vi "DMSC.main.vi"() -> ()   [LabVIEW 2014, in "DMSClient.lvlib"]
doc: "This CS tool subscribes to the following information of a CS controls domain.\n\n \"DOMAINNAME_Tasks@NODENAME\": A list of taks. Each task has a name, command line parameters and options. There is one service for each node.\n\nHistory: 16-FEB-2006, Dietrich Beck\n\nCopyright (C)\nGesellschaft für Schwerionenforschung, GSI\nPlanckstr. 1\n64291 Darmstadt\nGermany\n\nContact: D.Beck@gsi.de \n\nThis program is free software; you can redistribute it and/or modify it under the terms of the \nGNU General Public License as published by the Free Software Foundation; either version 2 of the license, or (at your option) any later version.\n\nThis program is distributed in the hope that it will be useful, but WITHOUT ANY WARRANTY; without even the implied warranty of MERCHANTABILITY or FITNESS FOR A PARTICULAR PURPOSE. See the GNU General License for more details (http://www.gnu.org).\n\nGesellschaft für Schwerionenforschung, GSI\nPlanckstr. 1, 64291 Darmstadt, Germany\nFor all questions and ideas contact D. Beck.\nLast update: 16-DEC-2005"
uses:
  DMSClient.lvlib
  DMSC.node_type.ctl
  DomainManagementUtils/DMSU.restart_mode.ctl
  DMSC.process_type.ctl
  CSlibraries/UtilityLib/UtilityLib.valueStatus.ctl
  CSlibraries-extern/DimLVEvent/LVDimInterface/LVDimInterface.dim service type.ctl
  <vilib>/Utility/config.llb/Read Key (Boolean).vi
  CSlibraries-extern/DimLVEvent/LVDimInterface/LVDimInterface.dic_info_service_notifier.vi
  CSlibraries-extern/DimLVEvent/LVDimInterface/LVDimInterface.lvlib
  CSlibraries-extern/DimLVEvent/NodeMon-LV/LVNodeInfo/LVNodeInfo.lvlib
  DomainManagementUtils/DMSUtils.lvlib
  CSlibraries/UtilityLib/UtilityLib.lvlib
  <vilib>/Utility/config.llb/NI_LVConfig.lvlib
panel:
  in  "PlaceHolder":bool
  out "myTasks":T1 {"processes"."restartMode" items=["UNKNOWN", "MANUAL", "ONCE", "ALWAYS", "KILL", "SHUTDOWN"]}
  in  "Messages":i32(listbox)
  in  "DMSSNode":string="DMSNode"
  in  "setDomain":bool
  in  "ProcessType":T3 {"restartMode" items=["UNKNOWN", "MANUAL", "ONCE", "ALWAYS", "KILL", "SHUTDOWN"]}
  in  "procTypeArr":T3[](array[typedef]) {"restartMode" items=["UNKNOWN", "MANUAL", "ONCE", "ALWAYS", "KILL", "SHUTDOWN"]}
  in  "DomainName":string="KSTest"
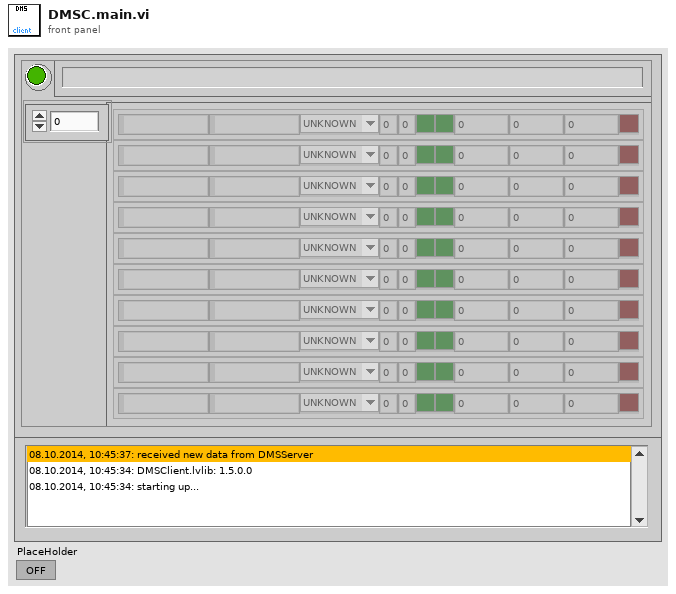
[diagram p1: front panel]
types:
  T1 = typedef "DMSClient.lvlib/DMSC.node_type.ctl" = cluster{"nodeName":string, "processes":cluster{"imageName":string, "argumentString":string, "restartMode":T2, "nOfRestart":i32, "resetRestartTimer":i32, "killOnExit":bool, "csSystem":bool, "PID":dbl, "PMem":dbl, "CPUTime":dbl, "startCnt":i32, "startTime":u32, "restartFailed":bool}[], "no link":bool}
  T2 = typedef "DMSUtils.lvlib/DMSU.restart_mode.ctl" = u16
  T3 = typedef "DMSClient.lvlib/DMSC.process_type.ctl" = cluster{"imageName":string, "argumentString":string, "restartMode":T2, "nOfRestart":i32, "resetRestartTimer":i32, "killOnExit":bool, "csSystem":bool, "PID":dbl, "PMem":dbl, "CPUTime":dbl, "startCnt":i32, "startTime":u32, "restartFailed":bool}
  T4 = cluster{"Command":enum16{"NewSystem", "DestroySystem", "SDSystem"}, "SystemName":string}
  T5 = enum32{"Invalid", "Standard", "Closed", "Hidden", "Minimized", "Maximized"}
  T6 = typedef "UtilityLib.lvlib/UtilityLib.valueStatus.ctl" = enum16{"no info available", "stand by/off", "on", "warning", "alarm/malfunction", "not implemented", "user action required", "important information", "system default", "control default", "indicator default", "button default"}
  T7 = enum16{"AddMessage", "AddErrorMessage", "GetMessages"}
  T8 = enum32{"invalid app kind", "Development System", "Run Time System", "Student Edition", "Embedded LabVIEW", "Evaluation", "Custom"}
  T9 = typedef "NI_LVConfig.lvlib/Config Data RefNum.ctl" = refnum<k1>
  T10 = typedef "LVDimInterface.lvlib/LVDimInterface.dim service type.ctl" = u16
  T11 = cluster{"imageName":string, "argumentString":string, "restartMode":T2, "nOfRestart":i32, "resetRestartTimer":i32, "killOnExit":bool, "csSystem":bool, "PID":dbl, "PMem":dbl, "CPUTime":dbl, "startCnt":i32, "startTime":u32, "restartFailed":bool}[]
  T12 = cluster{"imageName":string, "argumentString":string, "restartMode":T2, "nOfRestart":i32, "resetRestartTimer":i32, "killOnExit":bool, "csSystem":bool, "PID":dbl, "PMem":dbl, "CPUTime":dbl, "startCnt":i32, "startTime":u32, "restartFailed":bool}
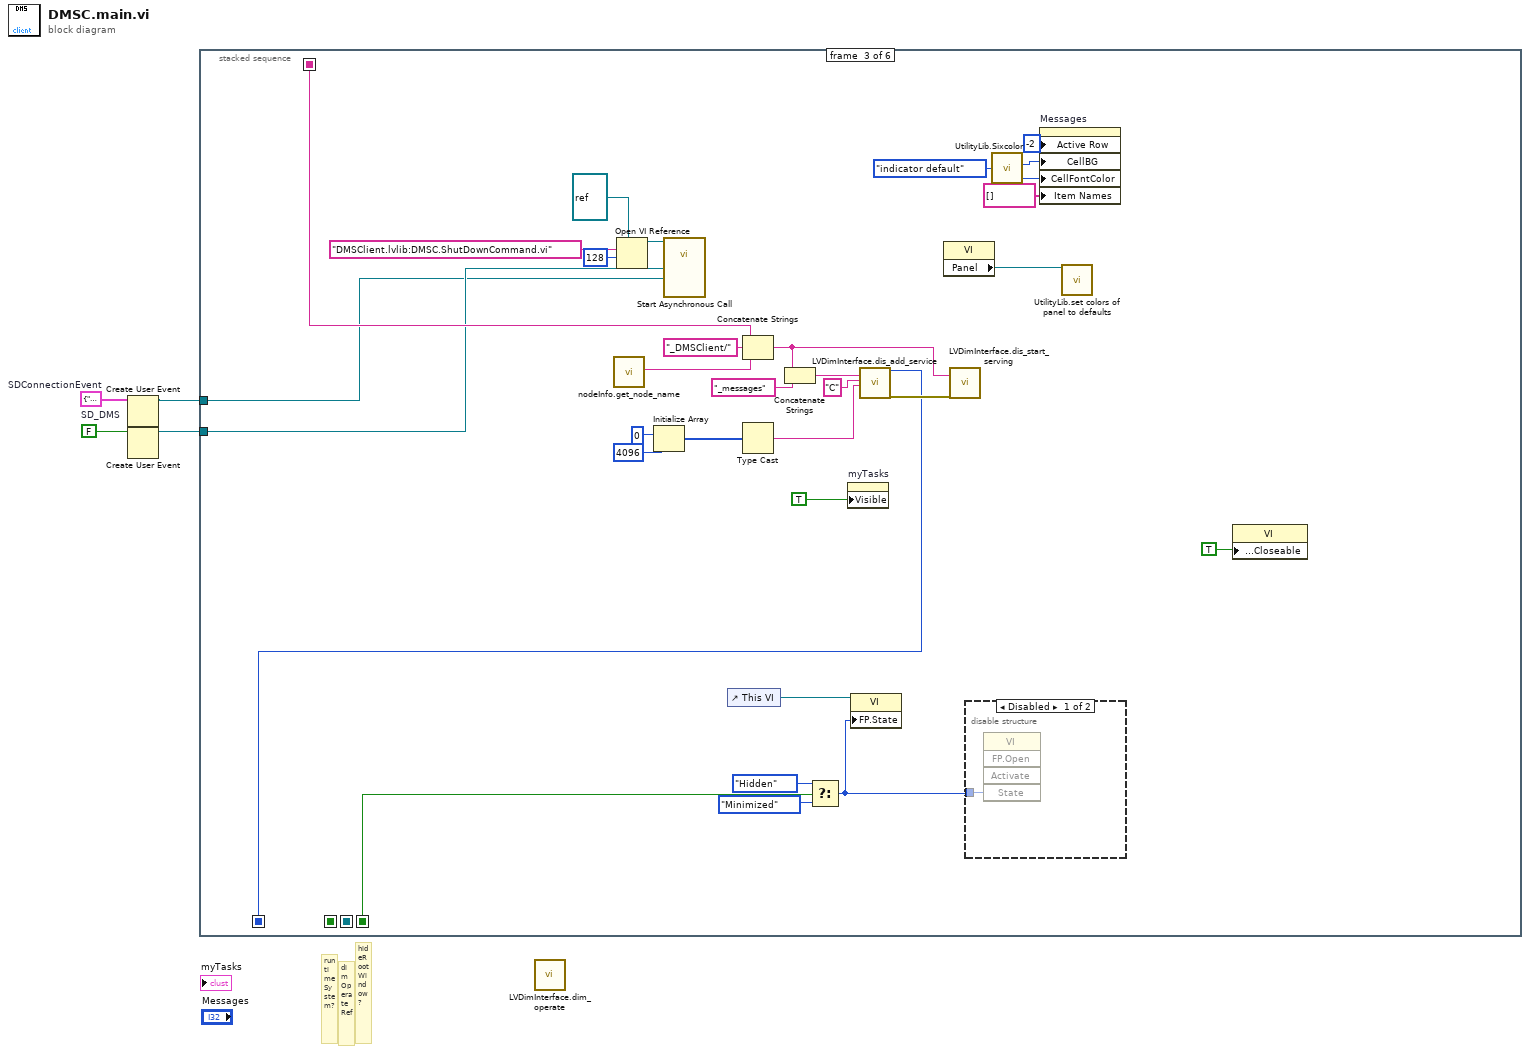
[diagram p0: block diagram]
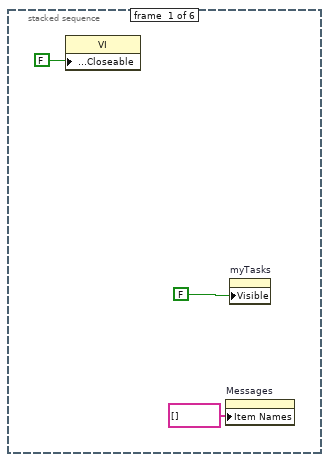
[diagram p2: hidden frame]
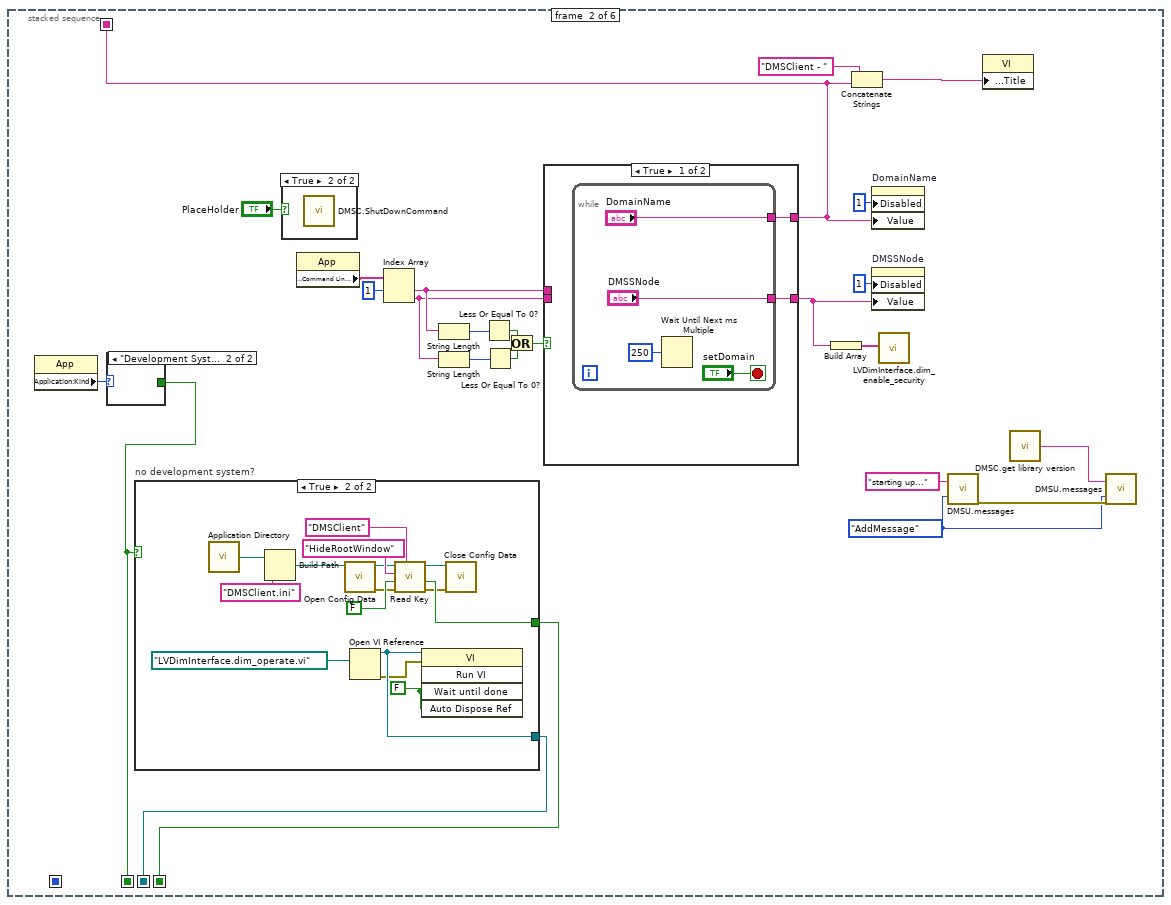
[diagram p3: hidden frame]
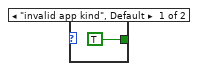
[diagram p5: hidden frame]
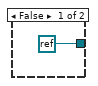
[diagram p6: hidden frame]
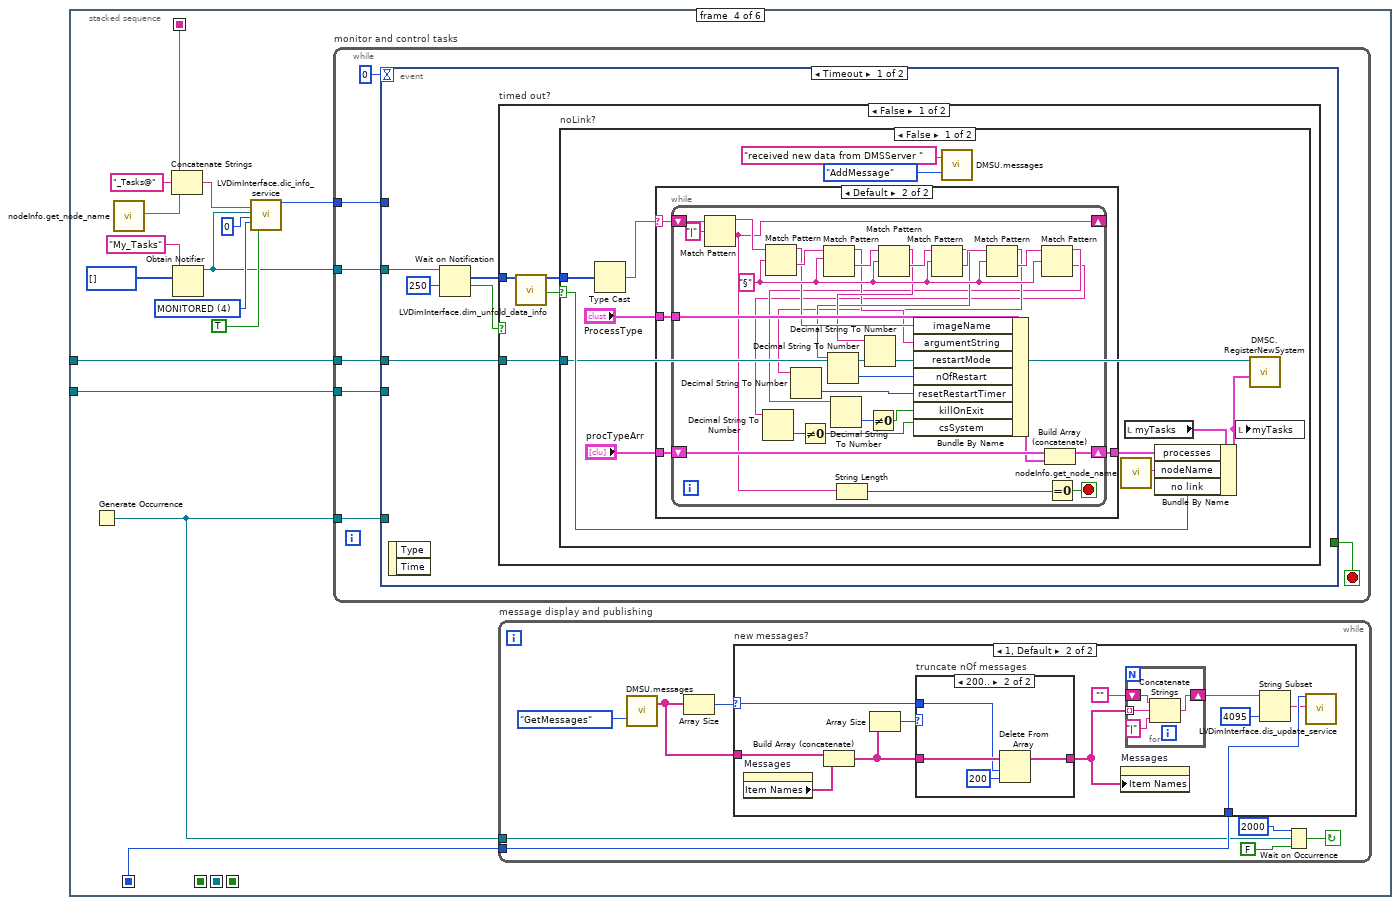
[diagram p9: hidden frame]
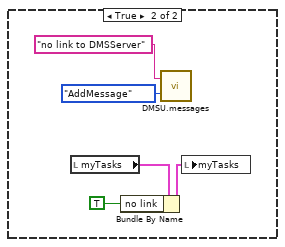
[diagram p13: hidden frame]
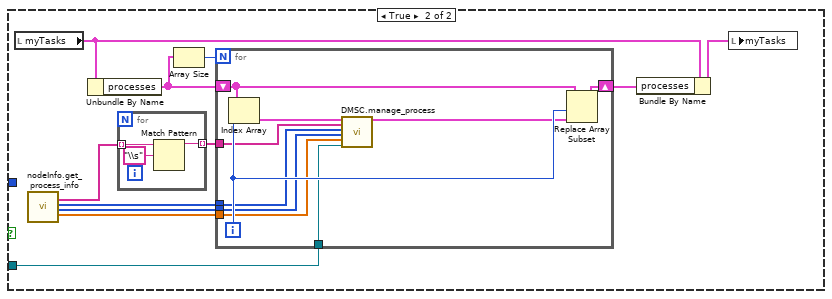
[diagram p14: hidden frame]
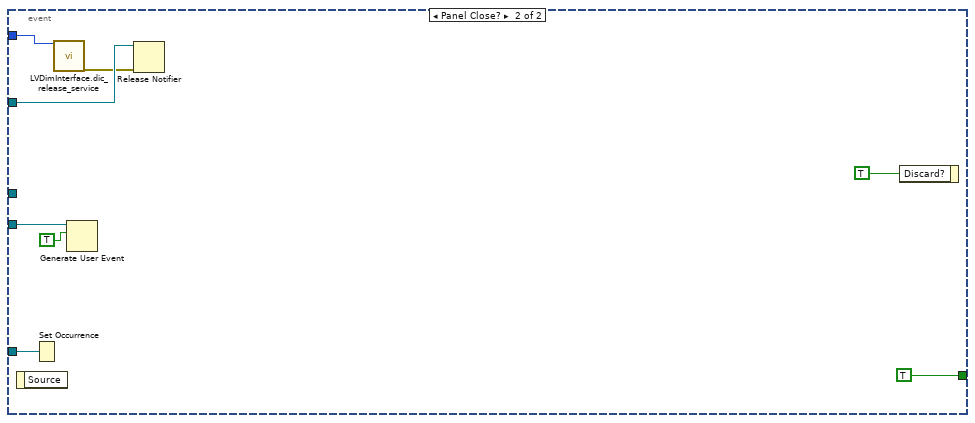
[diagram p15: hidden frame]
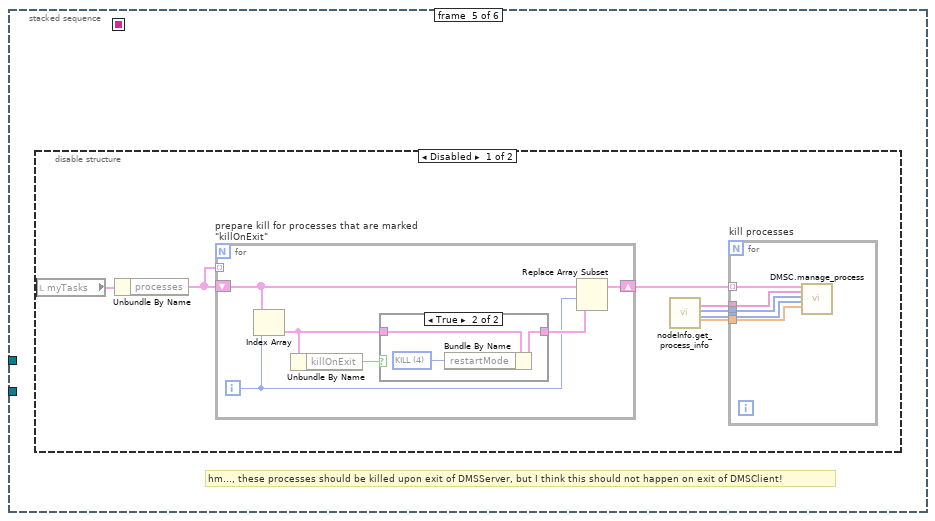
[diagram p16: hidden frame]
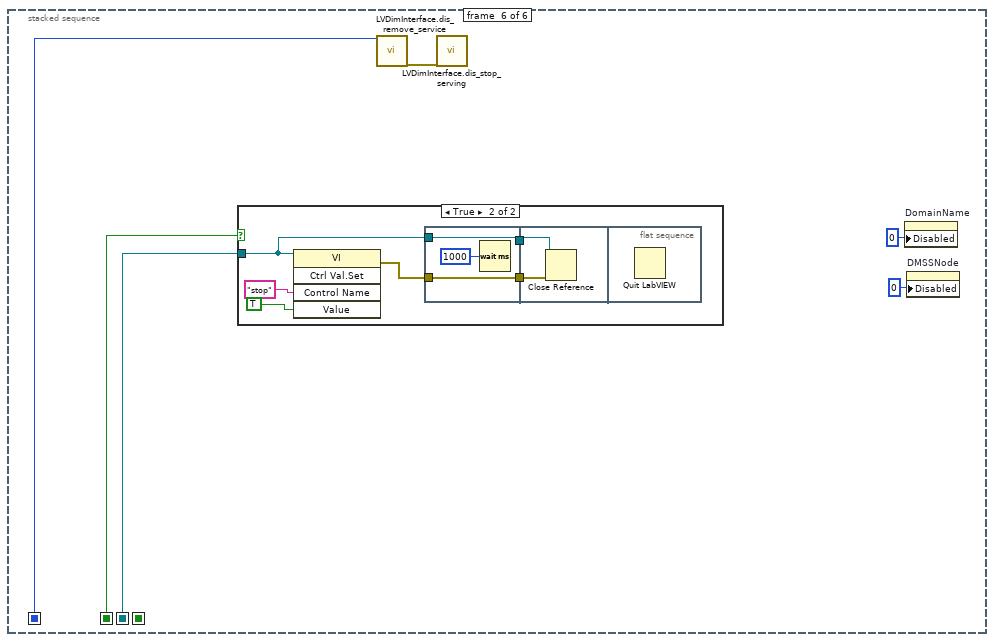
[diagram p19: hidden frame]
diagram:
  w3 = T4 {"Command"=enum."NewSystem", "SystemName"=""}  # SDConnectionEvent
  w4 = FALSE  # SD_DMS
  # "hideRootWindow?"
  # "dimOperateRef"
  # "runtimeSystem?"
  n1 = Create User Event(user event datatype=w3) -> (user event=w2:refnum<user-event>)  [unwired: 1 in, 1 out]
  n2 = Create User Event(user event datatype=w4) -> (user event=w1:refnum<user-event>)  [unwired: 1 in, 1 out]
  n3 = stacked-sequence {
    seq-local: [_ w15 _ _ _ _] -> [_ _ w76 w105 _ _]
    seq-local: [_ w17 _ _ _ _] -> [_ _ _ _ _ w256]
    seq-local: [_ w19 _ _ _ _] -> [_ _ _ _ _ w257]
    seq-local: [_ _ w77 _ _ _] -> [_ _ _ w94 _ w258]
    seq-local: [_ w12 _ _ _ _] -> [_ _ w64 _ _ _]
    tunnel: w2 -> [_ _ w60 w92 _ _]
    tunnel: w1 -> [_ _ w61 w91 _ _]
    frame #0 {
      n4 = property class="VI"("Front Panel.Closeable"=FALSE ("Front Panel Window:Closeable")) -> ()  [unwired: 2 in, 2 out]
      n5 = property on="Messages" class="LstBox (strict)"("Item Names"=string[] []) -> ()  [unwired: 2 in, 2 out]
      n6 = property on="myTasks" class="Clust (strict)"("Visible"=FALSE) -> ()  [unwired: 2 in, 2 out]
    }
    frame #1 {
      w9 = T7."AddMessage" ("Action")
      n7 = property on="Property Node" class="App"() -> ("Application:Kind"=w18:T8)  [unwired: 2 in, 2 out]
      n8 = case shown="\"Development System\"" w18 {
        tunnel: [TRUE _] -> w17
        frame "invalid app kind", Default {
        }
        frame "Development System" {
        }
      }
      n9 = case "no development system?" shown="True" w17 {
        tunnel: [refnum<k0> refnum ("Not a Refnum Constant") w47] -> w19
        tunnel: [_ w45] -> w12
        frame False {
        }
        frame True {
          w48 = FALSE ("Wait until done")
          n10 = call <vilib>:"Application Directory.vi"() -> ("Application Directory"=w35:path)
          n11 = Build Path(base path=w35, name or relative path="DMSClient.ini") -> (appended path=w36:path)
          n12 = call <vilib>:"Open Config Data.vi"("configuration file path"=w36) -> ("error out"=w38:errorcluster, "refnum"=w41:T9)  [unwired: 8 in, 1 out]
          n13 = Open VI Reference(vi path=path "LVDimInterface.dim_operate.vi") -> (vi reference=w47:refnum<vi>, error out=w46:errorcluster)  [unwired: 5 in]
          n14 = call-poly <vilib>:"Read Key.vi"("section"="DMSClient", "error in (no error)"=w38, "default value"=FALSE, "key"="HideRootWindow", "refnum"=w41) -> ("error out"=w37:errorcluster, "value"=w45:bool, "refnum out"=w40:T9)  [unwired: 3 in, 1 out]
          n15 = invoke on="Invoke Node" class="VI" method="Run VI"(reference=w47, error in=w46, "Wait until done"=w48, "Auto Dispose Ref"=w48) -> ()  [unwired: 1 in, 5 out]
          n16 = call <vilib>:"Close Config Data.vi"("error in (no error)"=w37, "refnum"=w40) -> ()  [unwired: 8 in, 2 out]
        }
      }
      n17 = case shown="True" "PlaceHolder" {
        frame False {
        }
        frame True {
          n18 = call "DMSC.ShutDownCommand.vi"() -> ()  [unwired: 20 in]
        }
      }
      n19 = property on="Property Node" class="App"() -> ("Application:Command Line Arguments"=w32:string[])  [unwired: 2 in, 2 out]
      n20 = Index Array(array=w32, index #1=1 ("index")) -> (element #1=w29:string, element #2=w23:string)  [unwired: 1 in]
      n21 = String Length(string=w29) -> (length=w30:i32)
      n22 = String Length(string=w23) -> (length=w27:i32)
      n23 = Less Or Equal To 0?(x=w30) -> (x <= 0?=w24:bool)
      n24 = Less Or Equal To 0?(x=w27) -> (x <= 0?=w25:bool)
      n25 = Or(x=w24, y=w25) -> (x .or. y?=w26:bool)
      n26 = case shown="True" w26 {
        tunnel: [w51 w57] -> w15
        tunnel: w29 -> [_ w57]
        tunnel: [w50 w56] -> w20
        tunnel: w23 -> [_ w56]
        frame True {
          n27 = while {
            tunnel: ["DomainName"] -> w51
            tunnel: ["DMSSNode"] -> w50
            stop <- "setDomain" stop-if-true
            n28 = Wait Until Next ms Multiple(millisecond multiple=u32 250) -> ()  [unwired: 1 out]
          }
        }
        frame False {
        }
      }
      n29 = Build Array(w20) -> (w21:string[])
      n30 = Concatenate Strings("DMSClient - " ("string"), w15) -> (w13:string)
      n31 = property on="DomainName" class="Str"("Disabled"=u8 1, "Value"=w15) -> ()  [unwired: 2 in, 2 out]
      n32 = property on="DMSSNode" class="Str"("Disabled"=u8 1, "Value"=w20) -> ()  [unwired: 2 in, 2 out]
      n33 = call "LVDimInterface.dim_enable_security.vi"("allowedNodes"=w21) -> ()  [unwired: 18 in, 1 out]
      n34 = call "DMSU.messages.vi"("message"="starting up...", "Action"=w9) -> ("error out"=w11:errorcluster)  [unwired: 16 in, 1 out]
      n35 = property on="Property Node" class="VI"("Front Panel.Title"=w13) -> ()  [unwired: 2 in, 2 out]
      n36 = call "DMSC.get library version.vi"() -> ("nameAndVersion"=w10:string)  [unwired: 1 in]
      n37 = call "DMSU.messages.vi"("message"=w10, "Action"=w9, "error in (no error)"=w11) -> ()  [unwired: 15 in, 2 out]
    }
    frame #2 {
      n38 = call "nodeInfo.get_node_name.vi"() -> ("nodeName"=w83:string)  [unwired: 18 in, 1 out]
      n39 = Open VI Reference(type specifier VI Refnum (for type only)=refnum<vi> refnum, vi path="DMSClient.lvlib:DMSC.ShutDownCommand.vi", options=128) -> (vi reference=w58:refnum<vi>)  [unwired: 3 in, 1 out]
      n40 = Initialize Array(u8 0, 4096 ("dimension size")) -> (w79:u8[])
      n41 = call-by-ref "Start Asynchronous Call"(reference=w58, "SD_DMS"=w61, "SDConnection Event"=w60) -> ()  [unwired: 19 in, 2 out]
      n42 = control-ref of="This VI"() -> (w66:refnum<vi>)
      n43 = Concatenate Strings(w76, "_DMSClient/" ("string"), w83) -> (w86:string)
      n44 = Type Cast(x=w79) -> (*(type *) &x=w78:string)  [unwired: 1 in]
      n45 = Concatenate Strings(w86, "_messages" ("string")) -> (w87:string)
      n46 = Select(t=T5."Hidden", s=w64, f=T5."Minimized" ("State")) -> (s? t:f=w65:T5)
      n47 = property on="myTasks" class="Clust (strict)"("Visible"=TRUE) -> ()  [unwired: 2 in, 2 out]
      n48 = property class="VI"(reference=w66, "FP.State"=w65) -> ()  [unwired: 1 in, 2 out]
      n49 = call "LVDimInterface.dis_add_service.vi"("serviceName"=w87, "typeDescriptor"="C", "data"=w78) -> ("my_serviceID"=w77:i32, "error out"=w85:errorcluster)  [unwired: 15 in]
      n50 = property on="Property Node" class="VI"() -> ("Panel"=w70:refnum<vi>)  [unwired: 2 in, 2 out]
      n51 = call "LVDimInterface.dis_start_serving.vi"("serverName"=w86, "error in (no error)"=w85) -> ()  [unwired: 16 in, 2 out]
      n52 = disable-structure shown="Disabled" {
        disable-tunnel: w65 -> [w90 _]
        frame Disabled {
          n53 = invoke on="Invoke Node" class="VI" method="FP.Open"("State"=w90) -> ()  [unwired: 4 in, 5 out]
        }
        frame Enabled {
        }
      }
      n54 = call "UtilityLib.Sixcolor.vi"("State"=UtilityLib.valueStatus."indicator default") -> ("elementBackground"=w74:u32, "elementText"=w73:u32)  [unwired: 2 in, 2 out]
      n55 = property on="Messages" class="LstBox (strict)"("Active Row"=-2 ("Active Row:Active Row Number"), "CellBG"=w74, "CellFontColor"=w73, "Item Names"=string[] []) -> ()  [unwired: 2 in, 2 out]
      n56 = call "UtilityLib.set colors of panel to defaults.vi"("Front Panel"=w70) -> ()  [unwired: 18 in, 1 out]
      n57 = property class="VI"("Front Panel.Closeable"=TRUE ("Front Panel Window:Closeable")) -> ()  [unwired: 2 in, 2 out]
    }
    frame #3 {
      w98 = T10 4 items=["ONCE_ONLY"=1, "TIMED"=2, "MONITORED"=4] ("serviceType")
      n58 = Generate Occurrence() -> (w93:refnum<k4>)
      n59 = call "nodeInfo.get_node_name.vi"() -> ("nodeName"=w104:string)  [unwired: 18 in, 1 out]
      n60 = Concatenate Strings(w105, "_Tasks@" ("string"), w104) -> (w102:string)
      n61 = Obtain Notifier(name (unnamed)="My_Tasks", notification data type=i8[] []) -> (notifier out=w95:refnum<notifier>)  [unwired: 2 in, 2 out]
      n62 = call-poly "LVDimInterface.dic_info_service.vi"("serviceName"=w102, "notifierRef"=w95, "timeout [s]"=0, "serviceType"=w98, "stamped"=TRUE) -> ("callBackID"=w96:i32)  [unwired: 13 in, 1 out]
      n63 = while "monitor and control tasks" {
        tunnel: w96 -> [w138]
        tunnel: w95 -> [w137]
        tunnel: w93 -> [w136]
        tunnel: w92 -> [w135]
        tunnel: w91 -> [w134]
        stop <- w139 stop-if-true
        n64 = event shown="[0] Timeout" {
          selector: _ -> [_ _]
          dyn-events: _ -> [_ _]
          timeout: 0 -> [_ _]
          tunnel: [_ TRUE ("Discard?")] -> w139
          tunnel: w138 -> [_ w233]
          tunnel: w137 -> [w145 w232]
          tunnel: w136 -> [_ w228]
          tunnel: w135 -> [w141 _]
          tunnel: w134 -> [_ w227]
          event Timeout {
            n65 = event-data() -> ()  [unwired: 1 in, 2 out]
            n66 = Wait on Notification(notifier=w145, timeout in ms (-1)=250) -> (notification=w144:i8[], timed out?=w143:bool)  [unwired: 2 in, 2 out]
            n67 = case "timed out?" shown="False" w143 {
              tunnel: w144 -> [w149 _]
              tunnel: w141 -> [w146 w202]
              frame False {
                n68 = call "LVDimInterface.dim_unfold_data_info.vi"("rawData"=w149) -> ("data"=w147:i8[], "no link"=w148:bool)  [unwired: 8 in, 9 out]
                n69 = case "noLink?" shown="False" w148 {
                  selector: w148 -> [w152 _]
                  tunnel: w147 -> [w161 _]
                  tunnel: w146 -> [w151 _]
                  frame False {
                    n70 = Type Cast(x=w161) -> (*(type *) &x=w153:string)  [unwired: 1 in]
                    n71 = case shown="Default" w153 {
                      selector: w153 -> [_ w163]
                      tunnel: "procTypeArr" -> [w162 w166]
                      tunnel: "ProcessType" -> [_ w165]
                      tunnel: [w162 w164] -> w156
                      frame "noTask" {
                      }
                      frame Default {
                        n72 = while {
                          shift-right: [w170] -> _
                          shift-left: w163 -> [w167]
                          shift-right: [w185] -> w164
                          shift-left: w166 -> [w186]
                          tunnel: w165 -> [w188]
                          stop <- w169 stop-if-true
                          w189 = "§" ("regular expression")
                          n73 = Match Pattern(string=w167, regular expression="|") -> (before substring=w195:string, after substring=w170:string)  [unwired: 1 in, 2 out]
                          n74 = Match Pattern(string=w195, regular expression=w189) -> (before substring=w187:string, after substring=w194:string)  [unwired: 1 in, 2 out]
                          n75 = Match Pattern(string=w194, regular expression=w189) -> (before substring=w179:string, after substring=w193:string)  [unwired: 1 in, 2 out]
                          n76 = String Length(string=w170) -> (length=w168:i32)
                          n77 = Match Pattern(string=w193, regular expression=w189) -> (before substring=w182:string, after substring=w192:string)  [unwired: 1 in, 2 out]
                          n78 = Decimal String To Number(string=w182) -> (number=w183:i32)  [unwired: 2 in, 1 out]
                          n79 = Match Pattern(string=w192, regular expression=w189) -> (before substring=w180:string, after substring=w191:string)  [unwired: 1 in, 2 out]
                          n80 = Decimal String To Number(string=w180) -> (number=w181:i32)  [unwired: 2 in, 1 out]
                          n81 = Match Pattern(string=w191, regular expression=w189) -> (before substring=w178:string, after substring=w190:string)  [unwired: 1 in, 2 out]
                          n82 = Decimal String To Number(string=w178) -> (number=w177:i32)  [unwired: 2 in, 1 out]
                          n83 = Match Pattern(string=w190, regular expression=w189) -> (before substring=w176:string, after substring=w171:string)  [unwired: 1 in, 2 out]
                          n84 = Decimal String To Number(string=w171) -> (number=w173:i32)  [unwired: 2 in, 1 out]
                          n85 = Not Equal To 0?(x=w173) -> (x != 0?=w172:bool)
                          n86 = Decimal String To Number(string=w176) -> (number=w175:i32)  [unwired: 2 in, 1 out]
                          n87 = Not Equal To 0?(x=w175) -> (x != 0?=w174:bool)
                          n88 = Bundle By Name(cluster=w188, "imageName"=w187, "argumentString"=w179, "restartMode"=w183, "nOfRestart"=w181, "resetRestartTimer"=w177, "killOnExit"=w174, "csSystem"=w172) -> (w184:T3)
                          n89 = Build Array (concatenate)(w186, w184) -> (w185:T3[])
                          n90 = Equal To 0?(x=w168) -> (x = 0?=w169:bool)
                        }
                      }
                    }
                    n91 = call "DMSU.messages.vi"("message"="received new data from DMSServer " ("string"), "Action"=T7."AddMessage") -> ()  [unwired: 16 in, 2 out]
                    n92 = call "nodeInfo.get_node_name.vi"() -> ("nodeName"=w157:string)  [unwired: 18 in, 1 out]
                    n93 = local read "myTasks"() -> (w158:T1)
                    n94 = Bundle By Name(cluster=w158, "processes"=w156, "nodeName"=w157, "no link"=w152) -> (w150:T1)
                    n95 = local write "myTasks"(w150) -> ()
                    n96 = call "DMSC.RegisterNewSystem.vi"("myTasks"=w150, "SDConnectionEvent"=w151) -> ()  [unwired: 10 in]
                  }
                  frame True {
                    n97 = local read "myTasks"() -> (w199:T1)
                    n98 = Bundle By Name(cluster=w199, "no link"=TRUE) -> (w198:T1)
                    n99 = call "DMSU.messages.vi"("message"="no link to DMSServer", "Action"=T7."AddMessage") -> ()  [unwired: 16 in, 2 out]
                    n100 = local write "myTasks"(w198) -> ()
                  }
                }
              }
              frame True {
                n101 = local read "myTasks"() -> (w207:T1)
                n102 = call "nodeInfo.get_process_info.vi"() -> ("procNames"=w203:string[], "procID"=w212:i32[], "procMemory"=w211:i32[], "procRuntime"=w210:dbl[])  [unwired: 14 in, 2 out]
                n103 = Unbundle By Name(w207) -> ("processes"=w208:T11)
                n104 = for {
                  tunnel: [w215] -> w204 mode=indexing
                  tunnel: w203 -> [w214] mode=indexing
                  n105 = Match Pattern(string=w214, regular expression="\\s") -> (before substring=w215:string)  [unwired: 1 in, 3 out]
                }
                n106 = Array Size(array=w208) -> (size(s)=w209:i32)
                n107 = for {
                  N: w209 -> [_]
                  tunnel: w204 -> [w220]
                  tunnel: w212 -> [w219]
                  tunnel: w211 -> [w218]
                  tunnel: w210 -> [w217]
                  shift-right: [w223] -> w206
                  shift-left: w208 -> [w224]
                  tunnel: w202 -> [w216]
                  i -> [w225]
                  n108 = Index Array(array=w224, index=w225) -> (element=w222:T12)
                  n109 = call "DMSC.manage_process.vi"("Process"=w222, "procNames"=w220, "procID"=w219, "procMemory"=w218, "procRuntime"=w217, "SDConnectionEvent"=w216) -> ("Process (out)"=w221:T3)  [unwired: 13 in]
                  n110 = Replace Array Subset(array=w224, new element=w221, index=w225) -> (w223:T11)
                }
                n111 = Bundle By Name(cluster=w207, "processes"=w206) -> (w205:T1)
                n112 = local write "myTasks"(w205) -> ()
              }
            }
          }
          event Panel Close? {
            n113 = event-data() -> ()  [unwired: 1 in, 1 out]
            n114 = Set Occurrence(w228) -> ()
            n115 = call "LVDimInterface.dic_release_service.vi"("callBackID"=w233) -> ("error out"=w231:errorcluster)  [unwired: 18 in]
            n116 = Generate User Event(user event=w227, event data cluster=TRUE ("SD_DMS")) -> ()  [unwired: 2 in, 2 out]
            n117 = Release Notifier(notifier=w232, error in (no error)=w231) -> ()  [unwired: 1 in, 3 out]
            n118 = event-data ("Event Filter Node")("Discard?"=TRUE) -> ()  [unwired: 1 in, 1 out]
          }
        }
      }
      n119 = while "message display and publishing" {
        tunnel: w93 -> [w106]
        tunnel: w94 -> [w107]
        stop <- w110 continue-if-true
        n120 = call "DMSU.messages.vi"("Action"=T7."GetMessages") -> ("messages"=w112:string[])  [unwired: 17 in, 1 out]
        n121 = Array Size(array=w112) -> (size(s)=w111:i32)
        n122 = case "new messages?" shown="1, Default" w111 {
          selector: w111 -> [_ w120]
          tunnel: w112 -> [_ w121]
          tunnel: w107 -> [_ w116]
          frame 0 {
          }
          frame 1, Default {
            n123 = property on="Messages" class="LstBox (strict)"() -> ("Item Names"=w124:string[])  [unwired: 2 in, 2 out]
            n124 = Build Array (concatenate)(w121, w124) -> (w122:string[])
            n125 = Array Size(array=w122) -> (size(s)=w123:i32)
            n126 = case "truncate nOf messages" shown="200.." w123 {
              tunnel: w122 -> [w129 w133]
              tunnel: w120 -> [_ w130]
              tunnel: [w129 w131] -> w119
              frame 0, Default {
              }
              frame 200.. {
                n127 = Delete From Array(array=w133, length=w130, index=200) -> (array with subset deleted=w131:string[])  [unwired: 1 out]
              }
            }
            n128 = property on="Messages" class="LstBox (strict)"("Item Names"=w119) -> ()  [unwired: 2 in, 2 out]
            n129 = for {
              tunnel: w119 -> [w127] mode=indexing
              shift-right: [w125] -> w118
              shift-left: "" ("Empty String Constant") -> [w128]
              n130 = Concatenate Strings(w128, w127, "|" ("string")) -> (w125:string)
            }
            n131 = String Subset(string=w118, length (rest)=4095 ("offset (0)")) -> (substring=w115:string)  [unwired: 1 in]
            n132 = call "LVDimInterface.dis_update_service.vi"("my_serviceID"=w116, "data"=w115) -> ()  [unwired: 15 in, 3 out]
          }
        }
        n133 = Wait on Occurrence(1:FALSE ("ignore previous (T)"), 2:w106, 3:2000 ("ms timeout (-1)")) -> (0:w110:bool)
      }
    }
    frame #4 {
      # "hm..., these processes should be killed upon exit of DMSServer, but I think this should not happen on exit of DMSClient!"
      n134 = disable-structure shown="Disabled" {
        frame Disabled {
          n135 = local read "myTasks"() -> (w240:T1)
          n136 = Unbundle By Name(w240) -> ("processes"=w234:T11)
          n137 = for "prepare kill for processes that are marked \"killOnExit\"" {
            shift-right: [w246] -> w239
            shift-left: w234 -> [w249]
            tunnel: w234 -> [_] mode=indexing
            i -> [w247]
            n138 = Index Array(array=w249, index=w247) -> (element=w250:T12)
            n139 = Unbundle By Name(w250) -> ("killOnExit"=w251:bool)
            n140 = case shown="True" w251 {
              tunnel: w250 -> [w252 w255]
              tunnel: [w252 w253] -> w248
              frame False {
              }
              frame True {
                w254 = T2 4 items=["UNKNOWN", "MANUAL", "ONCE", "ALWAYS", "KILL"] ("restartMode")
                n141 = Bundle By Name(cluster=w255, "restartMode"=w254) -> (w253:T12)
              }
            }
            n142 = Replace Array Subset(array=w249, new element=w248, index=w247) -> (w246:T11)
          }
          n143 = call "nodeInfo.get_process_info.vi"() -> ("procNames"=w238:string[], "procID"=w237:i32[], "procMemory"=w236:i32[], "procRuntime"=w235:dbl[])  [unwired: 14 in, 2 out]
          n144 = for "kill processes" {
            tunnel: w239 -> [w245] mode=indexing
            tunnel: w238 -> [w244]
            tunnel: w237 -> [w243]
            tunnel: w236 -> [w242]
            tunnel: w235 -> [w241]
            n145 = call "DMSC.manage_process.vi"("Process"=w245, "procNames"=w244, "procID"=w243, "procMemory"=w242, "procRuntime"=w241) -> ()  [unwired: 14 in, 1 out]
          }
        }
        frame Enabled {
        }
      }
    }
    frame #5 {
      n146 = case shown="True" w256 {
        tunnel: w257 -> [_ w264]
        frame False {
        }
        frame True {
          n147 = invoke on="Invoke Node" class="VI" method="Ctrl Val.Set"(reference=w264, "Control Name"="stop", "Value"=TRUE) -> (error out=w266:errorcluster)  [unwired: 2 in, 4 out]
          n148 = flat-sequence {
            tunnel: w264 -> [w269]
            tunnel: w266 -> [w270]
            tunnel: [w270] -> w263
            tunnel: [w269] -> w262
            tunnel: w263 -> [w272]
            tunnel: w262 -> [w271]
            frame #0 {
              n149 = Wait (ms)(milliseconds to wait=u32 1000) -> ()  [unwired: 1 out]
            }
            frame #1 {
              n150 = Close Reference(reference=w271, error in (no error)=w272) -> ()  [unwired: 1 out]
            }
            frame #2 {
              n151 = Quit LabVIEW() -> ()  [unwired: 1 in]
            }
          }
        }
      }
      n152 = call "LVDimInterface.dis_remove_service.vi"("my_serviceID"=w258) -> ("error out"=w259:errorcluster)  [unwired: 18 in]
      n153 = call "LVDimInterface.dis_stop_serving.vi"("error in (no error)"=w259) -> ()  [unwired: 18 in, 1 out]
      n154 = property on="DomainName" class="Str"("Disabled"=u8 0) -> ()  [unwired: 2 in, 2 out]
      n155 = property on="DMSSNode" class="Str"("Disabled"=u8 0) -> ()  [unwired: 2 in, 2 out]
    }
  }
  n156 = call "LVDimInterface.dim_operate.vi"() -> ()  [unwired: 20 in]
